vi "setXAxisConversionType.vi"(6 "Delay between send and receive [ms]":i32=100, 8 "error in (no error)":errorcluster, 10 "type":i32, 11 "CCD in":refnum<class "CCD.lvclass">) -> (0 "error out":errorcluster, 1 "ID":i32, 2 "results-JSON string":string, 3 "CCD out":refnum<class "CCD.lvclass">)   [LabVIEW 2023, in "CCD.lvclass"]
doc: "Sets the X-axis pixel conversion type to be used when retrieving the acquisition data with the ccd_getAcquisitionData command.\n\nNote: To use the parameters contained in the icl_settings.ini file, the ccd_setCenterWavelength command must be called first.\n\ntype Integer. The X-axis pixel conversion type to be used.\n0 = None (default)\n1 = CCD FIT parameters contained in the CCD firmware\n2 = Mono Wavelength parameters contained in the icl_settings.ini file"
uses:
  CCD.lvclass
  CCD.lvclass/CCD.ctl
  20f7d3bd-08ac-4524-9bed-df36c1da25a0.vi
  GenericDevice/GenericDevice.lvclass
  3e78960f-3857-40ea-b6b5-da67a5e4625c.vi
panel:
  # "Connector Pane"
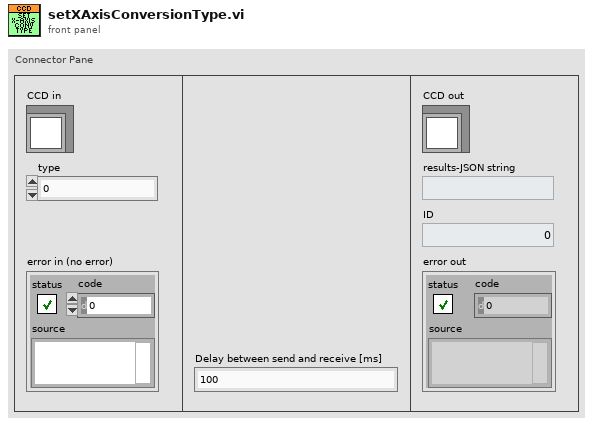
[diagram p1: front panel]
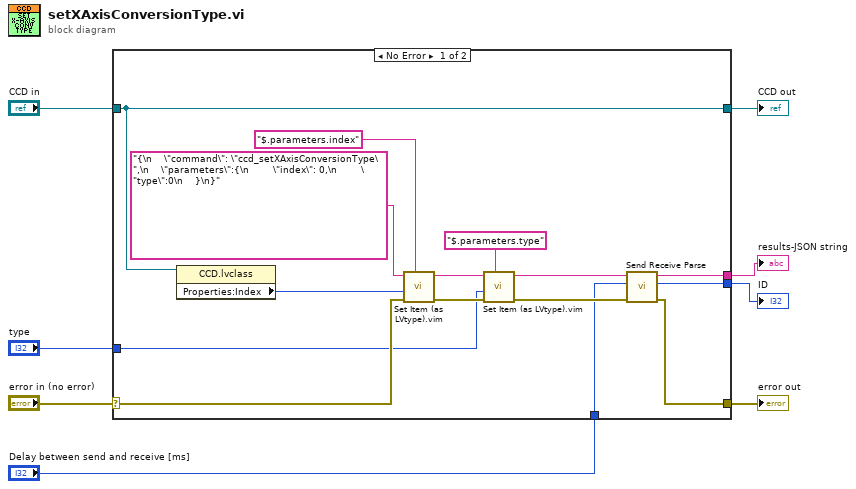
[diagram p0: block diagram]
diagram:
  n1 = case shown="No Error" "error in (no error)" {
    selector: "error in (no error)" -> [w19 w25]
    tunnel: [w14 w25] -> w7
    tunnel: [w21 w24] -> w5
    tunnel: "CCD in" -> [w21 w24]
    tunnel: [w13 _] -> w4
    tunnel: [w12 _] -> w3
    tunnel: "Delay between send and receive [ms]" -> [w10 _]
    tunnel: "type" -> [w9 _]
    frame No Error {
      n2 = property class="CCD.lvclass"(reference=w21) -> ("Properties:Index"=w20:i32)  [unwired: 1 in, 2 out]
      n3 = call "Set Item (as LVtype).vim"("$Path or Item Name"="$.parameters.index", "error in (no error)"=w19, "Anything"=w20, "JSON"="{\n    \"command\": \"ccd_setXAxisConversionType\",\n    \"parameters\":{\n        \"index\": 0,\n        \"type\":0\n    }\n}") -> ("error out"=w17:errorcluster, "<JSON>"=w18:string)  [unwired: 4 in, 1 out]
      n4 = call "Set Item (as LVtype).vim"("$Path or Item Name"="$.parameters.type", "error in (no error)"=w17, "Anything"=w9, "JSON"=w18) -> ("error out"=w16:errorcluster, "<JSON>"=w11:string)  [unwired: 4 in, 1 out]
      n5 = call "Send Receive Parse.vi"("error in"=w16, "Delay between send and receive [ms]"=w10, "<JSON>"=w11) -> ("error out"=w14:errorcluster, "ID"=w12:i32, "results-JSON string"=w13:string)  [unwired: 6 in]
    }
    frame Error {
    }
  }
  "error out" <- w7
  "CCD out" <- w5
  "results-JSON string" <- w4
  "ID" <- w3
